vi "Set-Trigger-mode.vi"(8 "error in (no error)":errorcluster, 10 "Trigger mode":T1=enum."Framegrabber timed (sync.)", 11 "PF_MV1-D1312-240 in":refnum<class "PF_MV1-D1312-240.lvclass">) -> (0 "error out":errorcluster, 3 "PF_MV1-D1312-240 out":refnum<class "PF_MV1-D1312-240.lvclass">)   [LabVIEW 2013, in "CameraVision.lvlib" / "PF_MV1-D1312-240.lvclass"]
uses:
  PF_MV1-D1312-240.lvclass
  Main/Acquisition/Trigger-modes.ctl
  Camera.lvclass/Camera.ctl
  <userlib>/Photonfocus Toolkit/_Public/SubVIs/pf_Set_Camera_Property_Mode.vi
  <userlib>/Photonfocus Toolkit/Photonfocus_Toolkit.lvlib
  Camera.lvclass
  Main/Acquisition/CV-Acquisition.lvclass
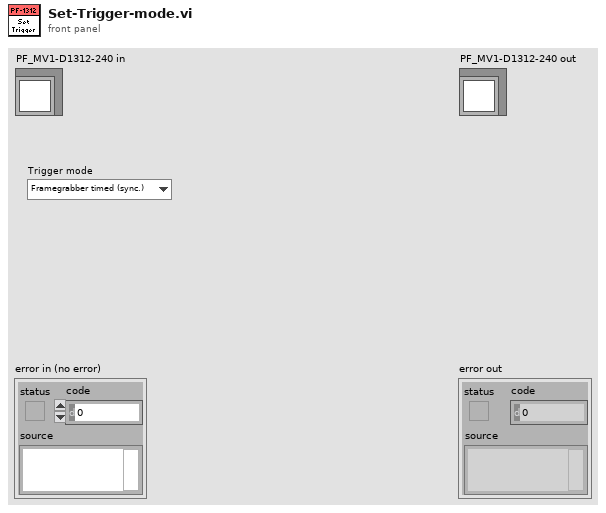
[diagram p1: front panel]
types:
  T1 = typedef "CameraVision.lvlib/CV-Acquisition.lvclass/Trigger-modes.ctl" = enum16{"Camera timed (not sync.)", "Framegrabber timed (sync.)", "Software timed (sync.)", "External timing (sync.)", "Manual (sync.)", "Gated - camera (not sync.)", "Gated - grabber (sync.)", "Gated - software (sync.)", "Gated - external (sync.)"}
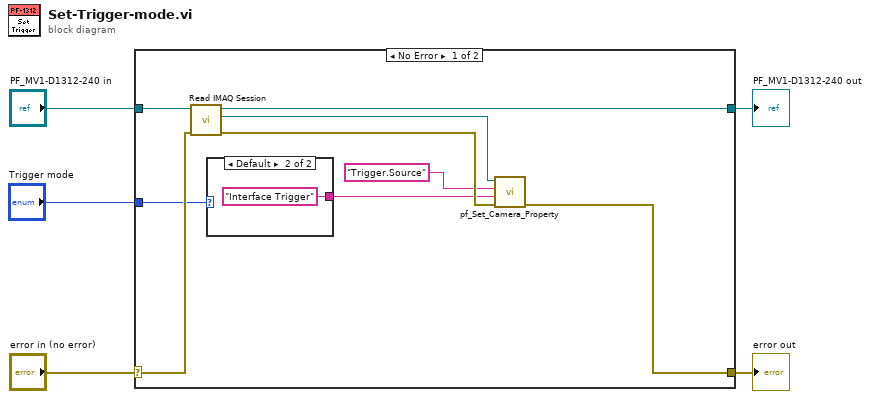
[diagram p0: block diagram]
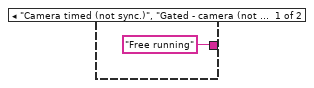
[diagram p2: hidden frame]
diagram:
  n1 = case shown="No Error" "error in (no error)" {
    selector: "error in (no error)" -> [w11 w18]
    tunnel: [w9 w18] -> w4
    tunnel: [w12 w17] -> w2
    tunnel: "PF_MV1-D1312-240 in" -> [w13 w17]
    tunnel: "Trigger mode" -> [w7 _]
    frame No Error {
      n2 = call "Read IMAQ Session.vi"("error in (no error)"=w11, "Camera in"=w13) -> ("error out"=w10:errorcluster, "IMAQ Session"=w14:refnum<k11>, "Camera out"=w12:refnum<class "PF_MV1-D1312-240.lvclass">)  [unwired: 7 in]
      n3 = case shown="Default" w7 {
        tunnel: ["Free running" "Interface Trigger"] -> w6
        frame "Camera timed (not sync.)", "Gated - camera (not sync.)" {
        }
        frame Default {
        }
      }
      n4 = call-poly <userlib>:"pf_Set_Camera_Property.vi"("error in (no error)"=w10, "Property Value"=w6, "Property Name"="Trigger.Source", "IMAQ Session in"=w14) -> ("error out"=w9:errorcluster)  [unwired: 5 in, 2 out]
    }
    frame Error {
    }
  }
  "error out" <- w4
  "PF_MV1-D1312-240 out" <- w2
